vi "Bookmark Project Provider Help.vi"   [LabVIEW 2015]
uses:
  <vilib>/Platform/browser.llb/Open URL in Default Browser (path).vi
  <vilib>/Platform/browser.llb/Open URL in Default Browser (string).vi
panel:
  # "Opening User Guide...."
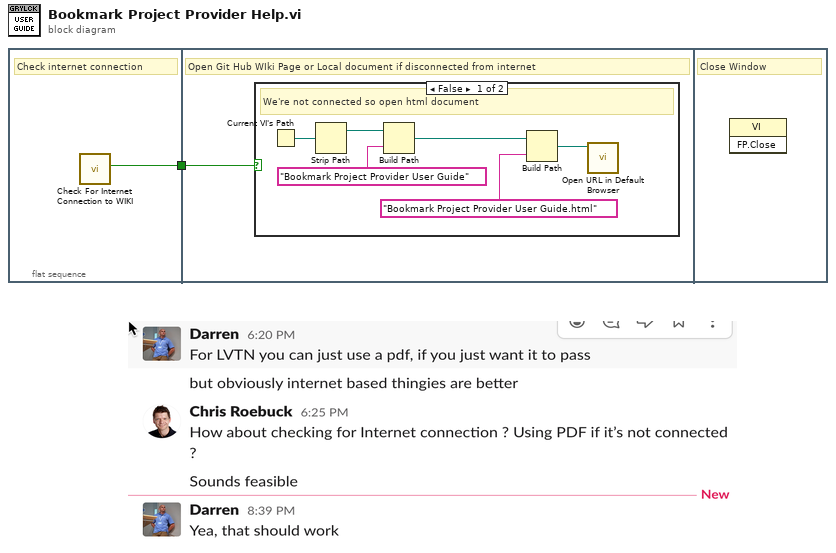
[diagram p0: block diagram]
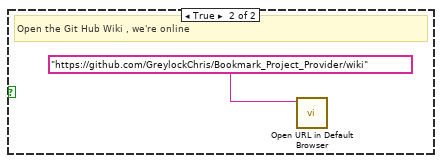
[diagram p2: hidden frame]
diagram:
  n1 = flat-sequence {
    tunnel: [w2] -> w1
    tunnel: w1 -> [w3]
    frame #0 {
      # "Check internet connection"
      n2 = call "Check For Internet Connection to WIKI.vi"() -> ("Connected to internet?"=w2:bool)  [unwired: 10 in, 1 out]
    }
    frame #1 {
      # "Open Git Hub WIki Page or Local document if disconnected from internet"
      n3 = case shown="False" w3 {
        frame False {
          # "We're not connected so open html document"
          n4 = Current VI's Path() -> (path=w9:path)
          n5 = Strip Path(path=w9) -> (stripped path=w8:path)  [unwired: 1 out]
          n6 = Build Path(base path=w8, name or relative path="Bookmark Project Provider User Guide") -> (appended path=w7:path)
          n7 = Build Path(base path=w7, name or relative path="Bookmark Project Provider User Guide.html") -> (appended path=w6:path)
          n8 = call-poly <vilib>:"Open URL in Default Browser.vi"("path"=w6) -> ()  [unwired: 5 in, 2 out]
        }
        frame True {
          # "Open the Git Hub Wiki , we're online"
          n9 = call-poly <vilib>:"Open URL in Default Browser.vi"("URL"="https://github.com/GreylockChris/Bookmark_Project_Provider/wiki") -> ()  [unwired: 5 in, 2 out]
        }
      }
    }
    frame #2 {
      # "Close Window"
      n10 = invoke class="VI" method="FP.Close"() -> ()  [unwired: 3 in, 3 out]
    }
  }
